vi "Dynamic Scoring Web.vi"(11 "LabVIEW Web Service Request":refnum<class "Web Request.lvclass">) -> ()   [LabVIEW 2013]
uses:
  <vilib>/wsapi/Web Request.lvclass
  ScoreEntry.ctl
panel:
  out "Value":string[](array[string])
  out "Key":string[](array[string])
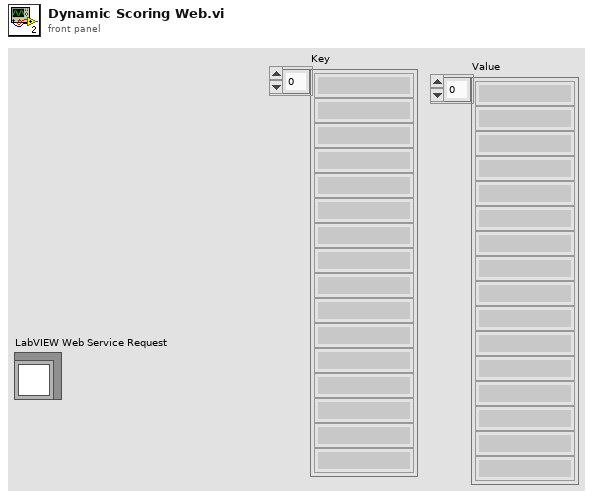
[diagram p1: front panel]
types:
  T1 = typedef "ScoreEntry.ctl" = cluster{"Elements":cluster{"Name":string, "Value":string}[], "Score":dbl}
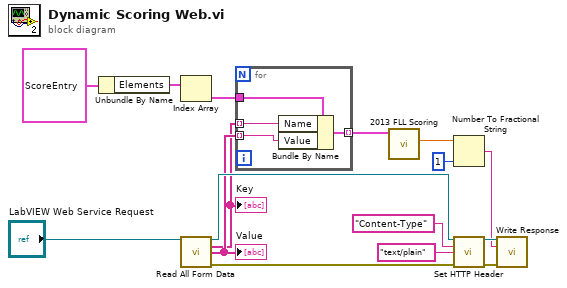
[diagram p0: block diagram]
diagram:
  n1 = Unbundle By Name(T1 {"Elements"=[{"Name"="CO2 Balls Touching/Within Reservoir Model", "Value"="-1"}, {"Name"="Money Ball Touching/Within Reservoir Model", "Value"="-1"}, {"Name"="3+ Red/White Citizens in Pink Grid Area", "Value"="-1"}, {"Name"="# Upright Levee Blocks touching ONLY GREEN shores", "Value"="-1"}, {"Name"="# Upright Levee Blocks Touching any RED shore", "Value"="-1"}, {"Name"="Levee Test was Performed", "Value"="-1"}, {"Name"="Levee Test Wheel Blocked by NonLevee", "Value"="-1"}, {"Name"="Flood Barrier in Up Position", "Value"="-1"}, {"Name"="Both Yellow Arrows Aligned", "Value"="-1"}, {"Name"="Team Robot Touching Only Yellow Grid Area", "Value"="-1"}, {"Name"="Both Insulation Touching Green Grid Area", "Value"="-1"}, {"Name"="Bicycle Touching Green Grid Area", "Value"="-1"}, {"Name"="Computer Touching Green Grid Area", "Value"="-1"}, {"Name"="House in Up Position", "Value"="-1"}, {"Name"="House Window Showing Black", "Value"="-1"}, {"Name"="House Window All The Way Open", "Value"="-1"}, {"Name"="3+ Black/White Scientists Touching Research Area", "Value"="-1"}, {"Name"="Money Ball Touching/Within Research Area Model", "Value"="-1"}, {"Name"="Polar Bear Touching/Within Research Area Model", "Value"="-1"}, {"Name"="Polar Bear Orientation (Sleeping/Upright)", "Value"="-1"}, {"Name"="Ice Core Pulled From Its Hole", "Value"="-1"}, {"Name"="Ice Buoy Upright and Within/Touching Research Area Model", "Value"="-1"}, {"Name"="Drilling Machine Touching/Within Research Area Model", "Value"="-1"}, {"Name"="Drill Assembly Completely Vertical", "Value"="-1"}, {"Name"="Team Robot Touching/Within Research Area Model", "Value"="-1"}, {"Name"="3+ Blue/Gray Leaders Touching Green Mountain/City Area", "Value"="-1"}, {"Name"="Ice Core in Base Area", "Value"="-1"}, {"Name"="Snowmobile Touching/Within Research Area Model", "Value"="-1"}], "Score"=0.0} ("Full Score Entry")) -> ("Elements"=w6:cluster{"Name":string, "Value":string}[])
  n2 = Index Array(array=w6) -> (element=w5:cluster{"Name":string, "Value":string})  [unwired: 1 in]
  n3 = call <vilib>:"Read All Form Data.vi"("LabVIEW Web Service Request"="LabVIEW Web Service Request") -> ("LabVIEW Web Service Request out"=w13:refnum<class "Web Request.lvclass">, "Key"=w8:string[], "Value"=w9:string[], "error out"=w12:errorcluster)  [unwired: 10 in, 1 out]
  "Key" <- w8
  "Value" <- w9
  n4 = for {
    tunnel: w9 -> [w18] mode=indexing
    tunnel: w8 -> [w19] mode=indexing
    tunnel: w5 -> [w20]
    tunnel: [w17] -> w4 mode=indexing
    n5 = Bundle By Name(cluster=w20, "Name"=w19, "Value"=w18) -> (w17:cluster{"Name":string, "Value":string})
  }
  n6 = call "2013 FLL Scoring.vi"("Array"=w4) -> ("Total Score"=w3:dbl)  [unwired: 9 in, 1 out]
  n7 = Number To Fractional String(number=w3, precision (6)=i16 1) -> (F-format string=w2:string)  [unwired: 2 in]
  n8 = call <vilib>:"Set HTTP Header.vi"("LabVIEW Web Service Request"=w13, "header"="Content-Type", "header value"="text/plain", "error in (no error)"=w12) -> ("LabVIEW Web Service Request out"=w11:refnum<class "Web Request.lvclass">, "error out"=w10:errorcluster)  [unwired: 10 in]
  n9 = call <vilib>:"Write Response.vi"("LabVIEW Web Service Request"=w11, "response string"=w2, "error in (no error)"=w10) -> ()  [unwired: 11 in, 2 out]
